vi "MultiLabelBinarizer.vi"(8 "error in (no error)":errorcluster caption="entrée d'erreur (pas d'erreur)", 11 "MultiLabelBinarizer":T1) -> (0 "error out":errorcluster, 3 "MultiLabelBinarizer.lvclass":refnum<class "MultiLabelBinarizer.lvclass">)   [LabVIEW 2020]
doc: "Transform between iterable of iterables and a multilabel format\n\nAlthough a list of sets or tuples is a very intuitive format for multilabel data, it is unwieldy to process. This transformer converts between this intuitive format and the supported multilabel format: a (samples x classes) binary matrix indicating the presence of a class label.\n\n\nParameters : \n\n- classes : array-like of shape [n_classes] (optional)\nIndicates an ordering for the class labels. All entries should be unique (cannot contain duplicate classes).\n\n- sparse_output : boolean (default: False),\nSet to true if output binary array is desired in CSR sparse format\n\n\nMethods: \n\n-Fit : Parameters : y : iterable of iterables\n A set of labels (any orderable and hashable object) for each sample. If the classes parameter is set, y will not be iterated.\n\n- Fit Transform : Fit the label sets binarizer and transform the given label sets\n\nParameters : y : iterable of iterables\n A set of labels (any orderable and hashable object) for each sample. If the classes parameter is set, y will not be iterated.\n\nReturns : y_indicator : array or CSR matrix, shape (n_samples, n_classes)\n A matrix such that y_indicator[i, j] = 1 iff classes_[j] is in y[i], and 0 otherwise.\n\n- Transform : Transform the given label sets\n\nParameters : y : iterable of iterables\n A set of labels (any orderable and hashable object) for each sample. If the classes parameter is set, y will not be iterated.\n\nReturns : y_indicator : array or CSR matrix, shape (n_samples, n_classes)\n A matrix such that y_indicator[i, j] = 1 iff classes_[j] is in y[i], and 0 otherwise."
uses:
  MultiLabelBinarizer.lvclass
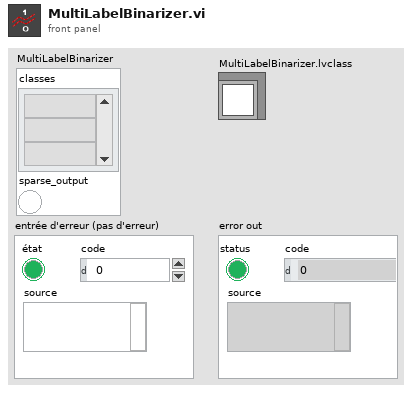
[diagram p1: front panel]
types:
  T1 = cluster{"classes":string[][], "sparse_output":bool}
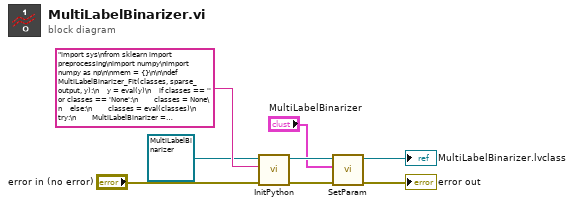
[diagram p0: block diagram]
diagram:
  n1 = call-dynamic "InitPython.vi"("error in (no error)"="error in (no error)", "Python Instruction"="import sys\nfrom sklearn import preprocessing\nimport numpy\nimport numpy as np\n\nmem = {}\n\n\ndef MultiLabelBinarizer_Fit(classes, sparse_output, y):\n    y = eval(y)\n    if classes == '' or classes == 'None':\n        classes = None\n    else:\n        classes = eval(classes)\n    try:\n        MultiLabelBinarizer = preprocessing.MultiLabelBinarizer(classes, sparse_output).fit(y)\n        mem['FitMultiLabelBinarizer'] = MultiLabelBinarizer\n        return str('OK')\n    except:\n        erreur = sys.exc_info()\n        typerr = u\"%s\" % (erreur[0])\n        typerr = typerr[typerr.find(\"'\")+1:typerr.rfind(\"'\")]\n        msgerr = u\"%s\" % (erreur[1])\n        message = str('/!\\\\ {0} : {1}'. format(typerr,msgerr))\n        return message \n    \ndef MultiLabelBinarizer_FitTransform(classes, sparse_output, y):\n    y = eval(y)\n    if classes == '' or classes == 'None':\n        classes = None\n    else:\n        classes = eval(classes)\n    try:\n        MultiLabelBinarizer = preprocessing.MultiLabelBinarizer(classes, sparse_output).fit_transform(y)\n        dtype = type(MultiLabelBinarizer)\n        if dtype == numpy.ndarray:\n            MultiLabelBinarizer = MultiLabelBinarizer.tolist()\n            return str(MultiLabelBinarizer) \n        else:\n            Mat = MultiLabelBinarizer.tocoo()\n            return str(list(zip(Mat.row, Mat.col, Mat.data)))\n    except:\n        erreur = sys.exc_info()\n        typerr = u\"%s\" % (erreur[0])\n        typerr = typerr[typerr.find(\"'\")+1:typerr.rfind(\"'\")]\n        msgerr = u\"%s\" % (erreur[1])\n        message = str('/!\\\\ {0} : {1}'. format(typerr,msgerr))\n        return message \n\ndef MultiLabelBinarizer_Transform(classes, sparse_output, y):\n    y = eval(y)\n    if classes == '' or classes == 'None':\n        classes = None\n    else:\n        classes = eval(classes)\n    try:\n        MultiLabelBinarizer = mem['FitMultiLabelBinarizer'].transform(y)\n        dtype = type(MultiLabelBinarizer)\n        if dtype == numpy.ndarray:\n            MultiLabelBinarizer = MultiLabelBinarizer.tolist()\n            return str(MultiLabelBinarizer) \n        else:\n            Mat = MultiLabelBinarizer.tocoo()\n            return str(list(zip(Mat.row, Mat.col, Mat.data)))\n    except:\n        erreur = sys.exc_info()\n        typerr = u\"%s\" % (erreur[0])\n        typerr = typerr[typerr.find(\"'\")+1:typerr.rfind(\"'\")]\n        msgerr = u\"%s\" % (erreur[1])\n        message = str('/!\\\\ {0} : {1}'. format(typerr,msgerr))\n        return message", "Scikit-learn en entrée"=refnum<class "MultiLabelBinarizer.lvclass"> refnum ("MultiLabelBinarizer.lvclass")) -> ("error out"=w5:errorcluster, "Scikit-learn en sortie"=w4:refnum<class "MultiLabelBinarizer.lvclass">)  [unwired: 7 in]
  n2 = call-dynamic "SetParam.vi"("error in (no error)"=w5, "MultiLabelBinarizer"="MultiLabelBinarizer", "MultiLabelBinarizer.lvclass"=w4) -> ("error out"=→"error out":errorcluster, "MultiLabelBinarizer.lvclass"=→"MultiLabelBinarizer.lvclass":refnum<class "MultiLabelBinarizer.lvclass">)  [unwired: 7 in]
